vi "getCustomerByJobOrLot.vi"(10 "Lot":string) -> (1 "Package":string, 3 "CustomerID":string)   [LabVIEW 2012]
uses:
  <vilib>/addons/database/Connection.llb/DB Tools Open Connec (Path).vi
  <vilib>/addons/database/Connection.llb/Conn Execute.vi
  <vilib>/addons/database/Recordset.llb/Rec Fetch Integer Data (R).vi
  <vilib>/addons/database/Recordset.llb/Rec Destroy - Connection.vi
  <vilib>/addons/database/Recordset.llb/Rec Fetch Recordset Data (R).vi
  <vilib>/addons/database/_DB Variant To Data/Database Variant To Data.xnode
  <vilib>/addons/database/NI_Database_API.lvlib
panel:
  out "error out 2":errorcluster
  out "before substring":string
  out "error out":errorcluster
  out "substring":string
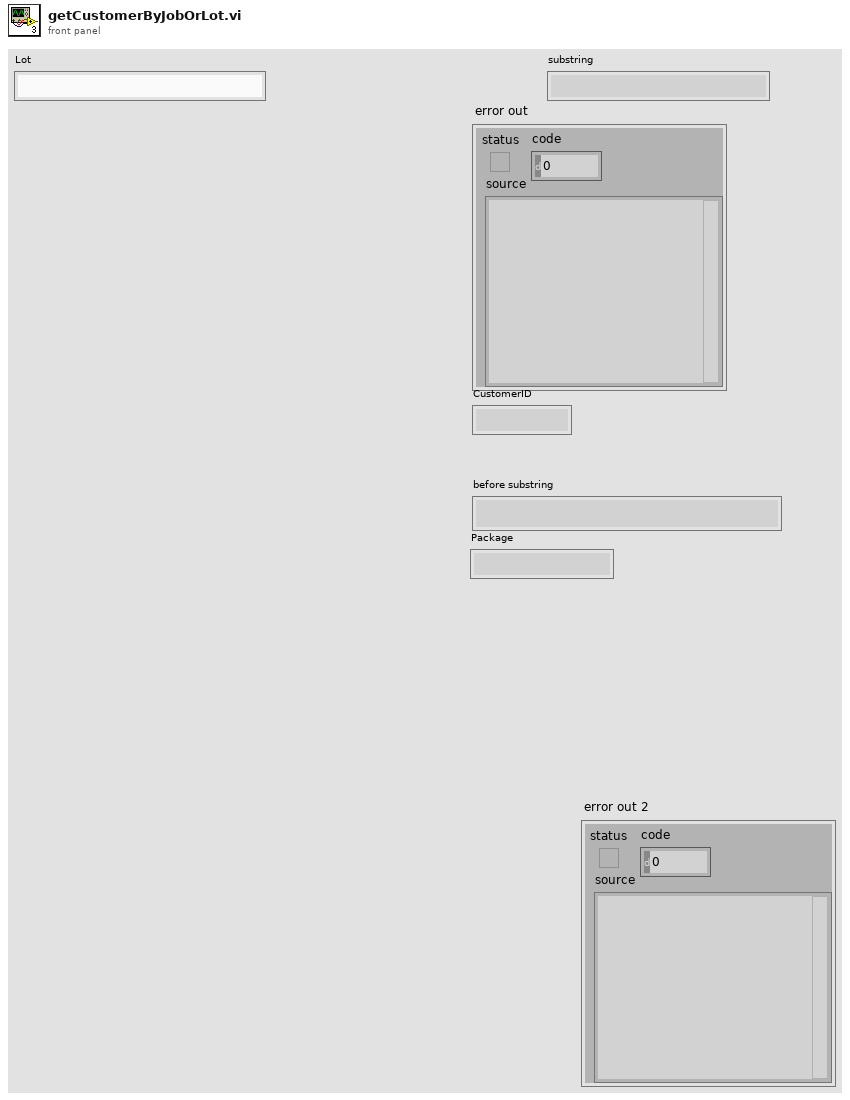
[diagram p1: front panel]
types:
  T1 = typedef "NI_Database_API.lvlib/Conn ObjectReference.ctl" = refnum<k1>
  T2 = typedef "NI_Database_API.lvlib/Rec ObjectReference.ctl" = refnum<k1>
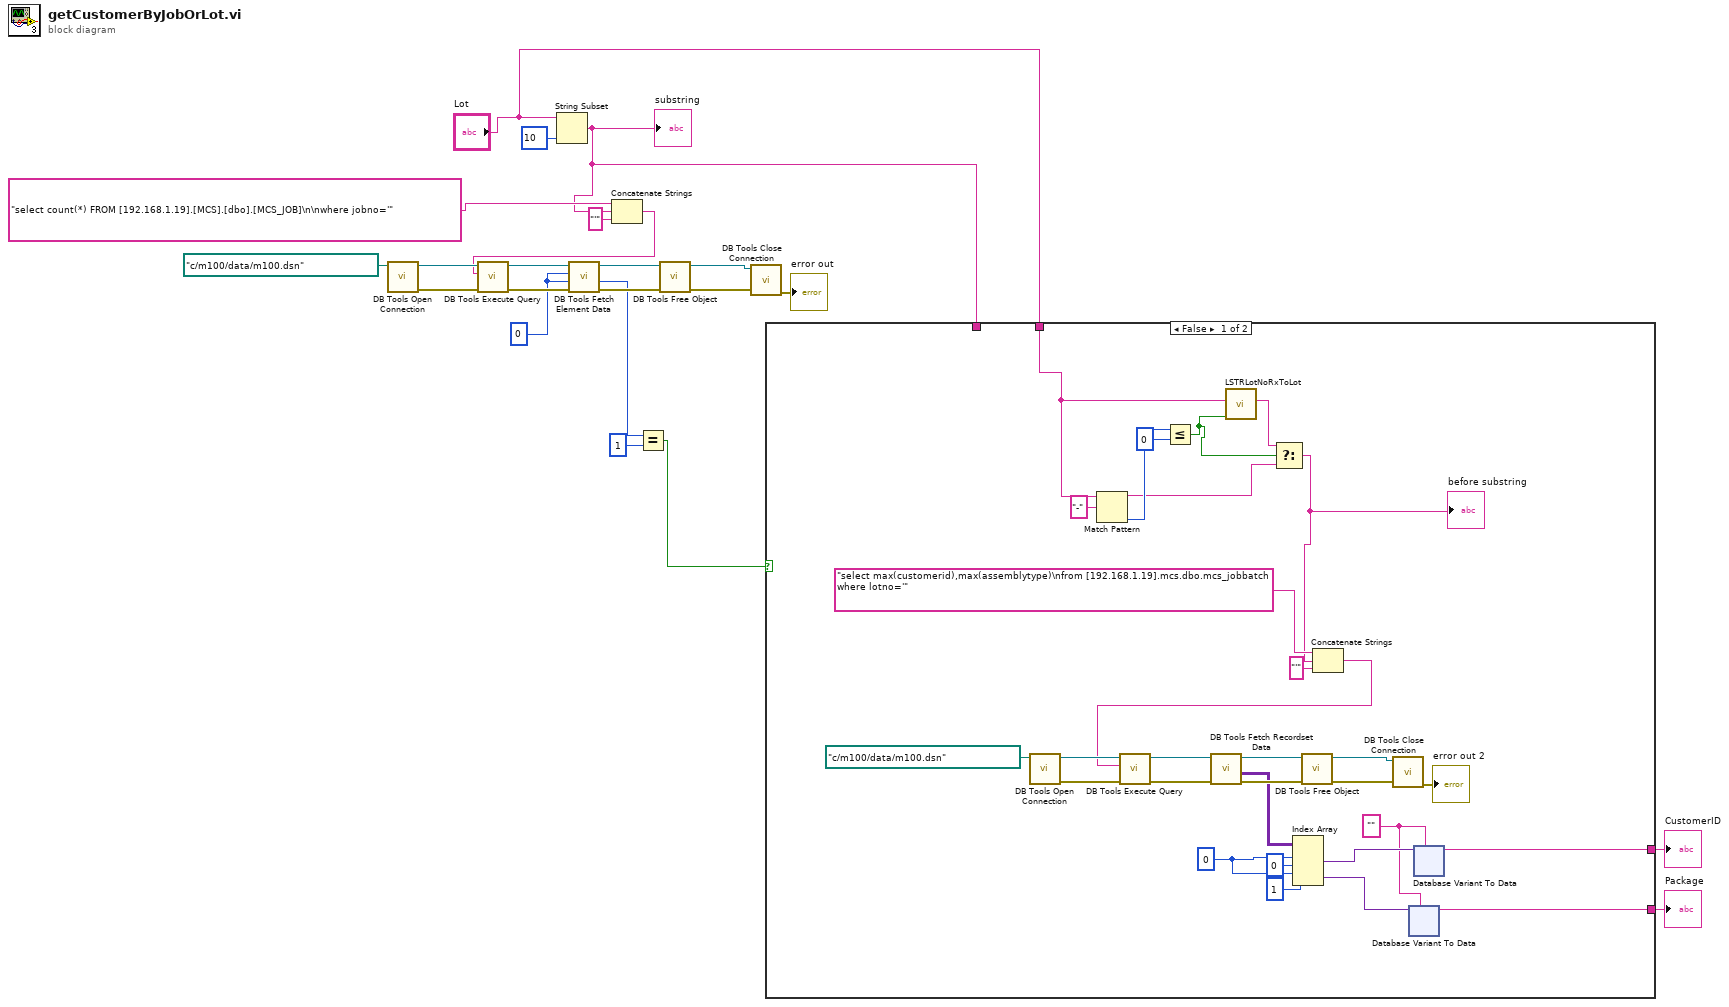
[diagram p0: block diagram]
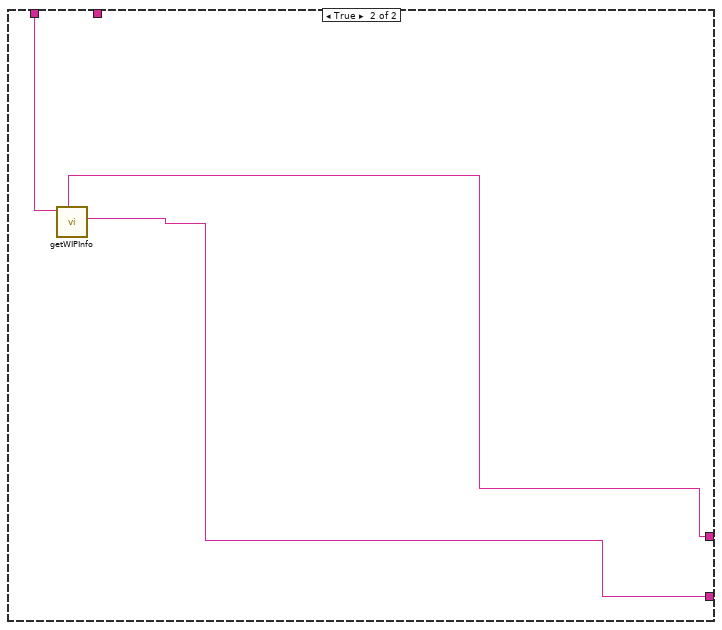
[diagram p2: hidden frame]
diagram:
  w11 = 0
  n1 = call-poly <vilib>:"DB Tools Open Connection.vi"("connection information"=path "c:/m100/data/m100.dsn") -> ("error out"=w18:errorcluster, "connection reference"=w21:T1)  [unwired: 7 in]
  n2 = String Subset(string="Lot", length (rest)=10 ("length (rest)")) -> (substring=w4:string)  [unwired: 1 in]
  "substring" <- w4
  n3 = Concatenate Strings("select count(*) FROM [192.168.1.19].[MCS].[dbo].[MCS_JOB]\n\nwhere jobno='" ("SQL query"), w4, "'" ("string")) -> (w12:string)
  n4 = call-poly <vilib>:"DB Tools Execute Query.vi"("error in (no error)"=w18, "SQL query"=w12, "connection reference"=w21) -> ("error out"=w17:errorcluster, "recordset reference"=w20:T2)  [unwired: 5 in]
  n5 = call-poly <vilib>:"DB Tools Fetch Element Data.vi"("error in (no error)"=w17, "type"=w11, "column index"=w11, "recordset reference"=w20) -> ("error out"=w16:errorcluster, "data"=w7:i32, "recordset reference out"=w19:T2)  [unwired: 3 in]
  n6 = Equal?(x=w7, y=1) -> (x = y?=w5:bool)
  n7 = call-poly <vilib>:"DB Tools Free Object.vi"("error in (no error)"=w16, "recordset reference"=w19) -> ("error out"=w9:errorcluster, "connection reference"=w10:T1)  [unwired: 8 in]
  n8 = call <vilib>:"DB Tools Close Connection.vi"("error in (no error)"=w9, "connection reference"=w10) -> ("error out"=→"error out":errorcluster)  [unwired: 5 in]
  n9 = case shown="False" w5 {
    tunnel: w4 -> [_ w119]
    tunnel: "Lot" -> [w27 _]
    tunnel: [w33 w117] -> w2
    tunnel: [w30 w118] -> w1
    frame False {
      w34 = 0 ("disabled index (row)")
      w31 = ""
      n10 = call-poly <vilib>:"DB Tools Open Connection.vi"("connection information"=path "c:/m100/data/m100.dsn") -> ("error out"=w48:errorcluster, "connection reference"=w51:T1)  [unwired: 7 in]
      n11 = Match Pattern(string=w27, regular expression="-") -> (before substring=w25:string, offset past match=w29:i32)  [unwired: 1 in, 2 out]
      n12 = Less Or Equal?(x=w29, y=0) -> (x <= y?=w26:bool)
      n13 = call "LSTRLotNoRxToLot.vi"("Boolean"=w26, "String"=w27) -> ("before match"=w23:string)  [unwired: 9 in]
      n14 = Select(t=w23, s=w26, f=w25) -> (s? t:f=w24:string)
      "before substring" <- w24
      n15 = Concatenate Strings("select max(customerid),max(assemblytype)\nfrom [192.168.1.19].mcs.dbo.mcs_jobbatch where lotno='" ("SQL query"), w24, "'" ("string")) -> (w39:string)
      n16 = call-poly <vilib>:"DB Tools Execute Query.vi"("error in (no error)"=w48, "SQL query"=w39, "connection reference"=w51) -> ("error out"=w47:errorcluster, "recordset reference"=w50:T2)  [unwired: 5 in]
      n17 = call-poly <vilib>:"DB Tools Fetch Recordset Data.vi"("error in (no error)"=w47, "recordset reference"=w50) -> ("error out"=w46:errorcluster, "recordset data"=w38:variant[][], "recordset reference out"=w49:T2)  [unwired: 3 in]
      n18 = Index Array(array=w38, index (row) #1=w34, index (col) #1=0 ("disabled index (col)"), index (row) #2=w34, index (col) #2=1 ("index (col)")) -> (element #1=w35:variant, element #2=w32:variant)
      n19 = call-poly <vilib>:"DB Tools Free Object.vi"("error in (no error)"=w46, "recordset reference"=w49) -> ("error out"=w43:errorcluster, "connection reference"=w44:T1)  [unwired: 8 in]
      n20 = call <vilib>:"DB Tools Close Connection.vi"("error in (no error)"=w43, "connection reference"=w44) -> ("error out"=→"error out 2":errorcluster)  [unwired: 5 in]
      n21 = xnode "Database Variant To Data"("database variant"=w32, "type"=w31) -> ("data"=w30:string)  [unwired: 1 in, 1 out]
      n22 = xnode "Database Variant To Data"("database variant"=w35, "type"=w31) -> ("data"=w33:string)  [unwired: 1 in, 1 out]
    }
    frame True {
      n23 = call "getWIPInfo.vi"("Lotno"=w119) -> ("Package"=w118:string, "CustomerID"=w117:string)  [unwired: 4 in, 5 out]
    }
  }
  "CustomerID" <- w2
  "Package" <- w1
